vi "int 32 to MSB LSB.vi"(11 "Signed 32 Bit Int":i32) -> (2 "LSB NUM":dbl, 3 "MSB NUM":dbl)   [LabVIEW 2014]
panel:
  out "LSB String":string
  out "MSB String":string
  out "Original String":string
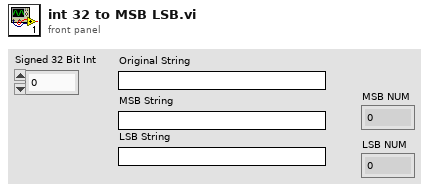
[diagram p1: front panel]
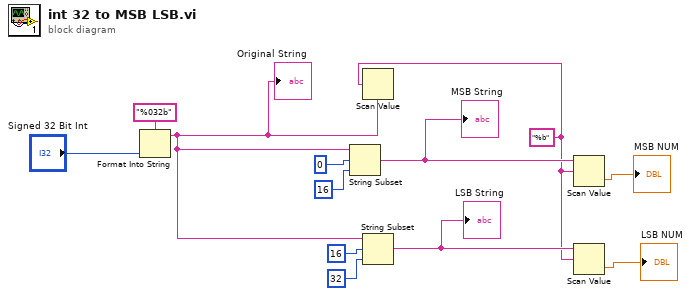
[diagram p0: block diagram]
diagram:
  w2 = "%b"
  n1 = Format Into String(format string="%032b", "Signed 32 Bit Int") -> (resulting string=w3:string)  [unwired: 2 in, 1 out]
  "Original String" <- w3
  n2 = String Subset(string=w3, offset (0)=0, length (rest)=16) -> (substring=w5:string)
  "MSB String" <- w5
  n3 = Scan Value(string=w3, format string=w2) -> (value=w1:dbl)  [unwired: 1 in, 1 out]
  n4 = String Subset(string=w3, offset (0)=16, length (rest)=32) -> (substring=w4:string)
  "LSB String" <- w4
  n5 = Scan Value(string=w5, format string=w2) -> (value=→"MSB NUM":dbl)  [unwired: 1 in, 1 out]
  n6 = Scan Value(string=w4, format string=w2) -> (value=→"LSB NUM":dbl)  [unwired: 1 in, 1 out]
